vi "ConfigSMU.vi"(8 "error in (no error)":errorcluster, 10 "gRPCid":T4, 11 "ctet_smu":T1) -> (0 "error out":errorcluster, 3 "ctet_smu out":T1)   [LabVIEW 2019, in "ctet_smu User Library.lvlib"]
uses:
  ctet_smu User Library.lvlib
  Servers/ctet_smu/gRPC lvSupport/Server API/typeDefs/grpcId.ctl
  Types/ctet_smu.ctl
  Servers/ctet_smu/ctet_smu Class/RPC Messages/measurementservice_SMUConfigResponse/measurementservice_SMUConfigResponse_Data.ctl
  Servers/ctet_smu/ctet_smu Class/RPC Messages/measurementservice_ErrorOut/measurementservice_ErrorOut_Data.ctl
  Servers/ctet_smu/ctet_smu Class/ctet_smu.lvclass
  Servers/ctet_smu/gRPC lvSupport/gprc-lvsupport.lvlib
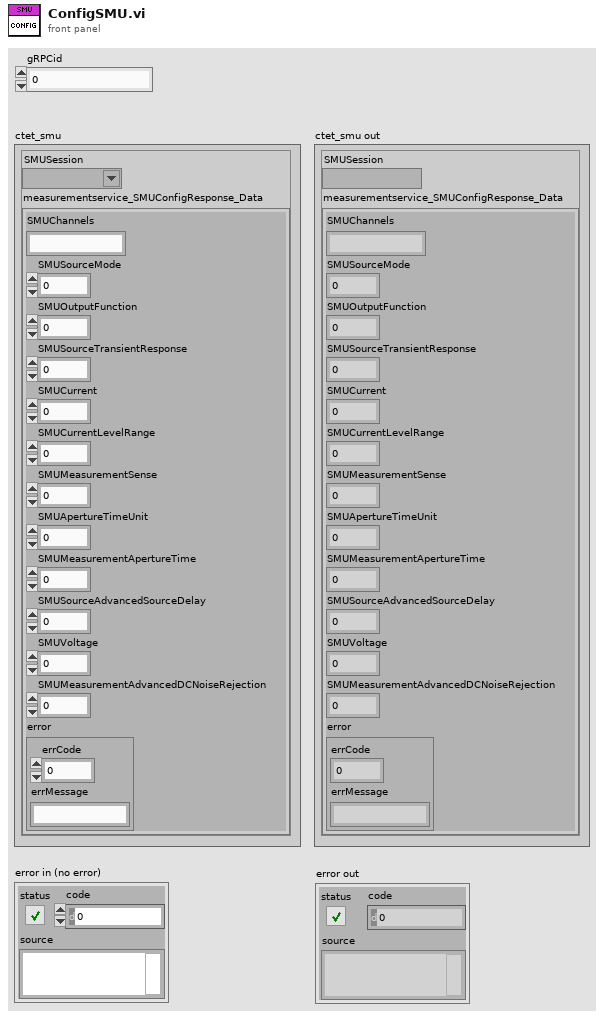
[diagram p1: front panel]
types:
  T1 = typedef "ctet_smu User Library.lvlib/ctet_smu.ctl" = cluster{"SMUSession":refnum<k15>, "measurementservice_SMUConfigResponse_Data":T2}
  T2 = typedef "ctet_smu.lvlib/ctet_smu.lvclass/measurementservice_SMUConfigResponse_Data.ctl" = cluster{"SMUChannels":string, "SMUSourceMode":i64, "SMUOutputFunction":i64, "SMUSourceTransientResponse":i64, "SMUCurrent":dbl, "SMUCurrentLevelRange":dbl, "SMUMeasurementSense":i64, "SMUApertureTimeUnit":i64, "SMUMeasurementApertureTime":dbl, "SMUSourceAdvancedSourceDelay":dbl, "SMUVoltage":dbl, "SMUMeasurementAdvancedDCNoiseRejection":i64, "error":T3}
  T3 = typedef "ctet_smu.lvlib/ctet_smu.lvclass/measurementservice_ErrorOut_Data.ctl" = cluster{"errCode":i64, "errMessage":string}
  T4 = typedef "ctet_smu.lvlib/gprc-lvsupport.lvlib/grpcId.ctl" = u64
  T5 = typedef "ctet_smu.lvlib/ctet_smu.lvclass/measurementservice_SMUConfigRequest_Data.ctl" = cluster{"SMUChannels":string, "SMUSourceMode":i64, "SMUOutputFunction":i64, "SMUSourceTransientResponse":i64, "SMUCurrent":dbl, "SMUCurrentLevelRange":dbl, "SMUMeasurementSense":i64, "SMUApertureTimeUnit":i64, "SMUMeasurementApertureTime":dbl, "SMUSourceAdvancedSourceDelay":dbl, "SMUVoltage":dbl, "SMUMeasurementAdvancedDCNoiseRejection":i64}
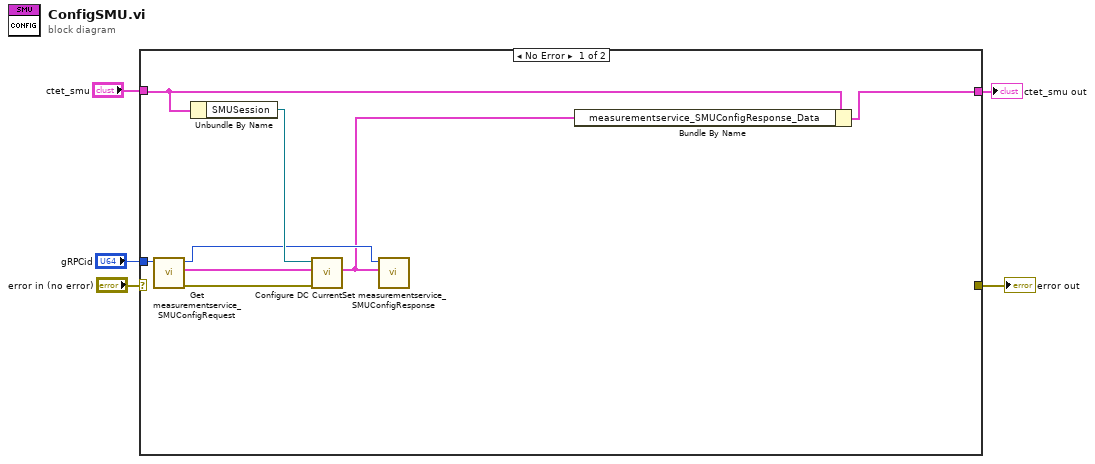
[diagram p0: block diagram]
diagram:
  n1 = case shown="No Error" "error in (no error)" {
    selector: "error in (no error)" -> [_ w15]
    tunnel: [_ w15] -> w5
    tunnel: "gRPCid" -> [w13 _]
    tunnel: "ctet_smu" -> [w11 w14]
    tunnel: [w8 w14] -> w1
    frame No Error {
      n2 = call "Get measurementservice_SMUConfigRequest.vi"("gRPCid"=w13) -> ("error out"=w9:errorcluster, "Message Data"=w12:T5, "gRPCid out"=w7:T4)  [unwired: 8 in]
      n3 = Unbundle By Name(w11) -> ("SMUSession"=w10:refnum<k15>)
      n4 = call "Configure DC Current.vi"("error in (no error)"=w9, "measurementservice_SMUConfigRequest_Data"=w12, "SMUSession"=w10) -> ("measurementservice_SMUConfigResponse_Data"=w6:T2)  [unwired: 7 in, 1 out]
      n5 = call "Set measurementservice_SMUConfigResponse.vi"("Message Data"=w6, "gRPCid"=w7) -> ()  [unwired: 9 in, 1 out]
      n6 = Bundle By Name(cluster=w11, "measurementservice_SMUConfigResponse_Data"=w6) -> (w8:T1)
    }
    frame Error {
    }
  }
  "error out" <- w5
  "ctet_smu out" <- w1
